vi "Day12-create_map.vi"(11 "string array":string[](array[string])) -> (3 "Map":map{string, string[]}(c390))   [LabVIEW 2021]
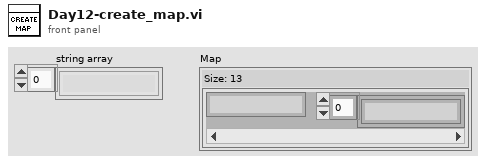
[diagram p1: front panel]
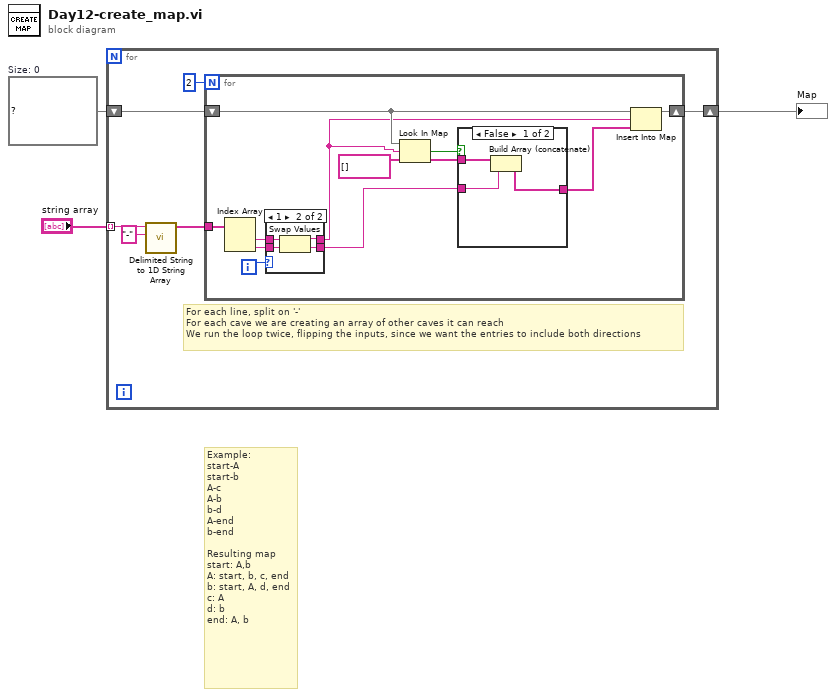
[diagram p0: block diagram]
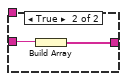
[diagram p3: hidden frame]
diagram:
  w2 = map{string, string[]} {}  # Size: 0
  # "Example:\nstart-A\nstart-b\nA-c\nA-b\nb-d\nA-end\nb-end\n\nResulting map\nstart: A,b\nA: start, b, c, end\nb: start, A, d, end\nc: A\nd: b\nend: A, b"
  n1 = for {
    tunnel: "string array" -> [w9] mode=indexing
    shift-right: [w6] -> w3
    shift-left: w2 -> [w7]
    # "For each line, split on '-'\nFor each cave we are creating an array of other caves it can reach\nWe run the loop twice, flipping the inputs, since we want the entries to include both directions"
    n2 = call <vilib>:"Delimited String to 1D String Array.vi"("delimiter"="-", "delimited string"=w9) -> ("string array"=w5:string[])  [unwired: 9 in]
    n3 = for {
      N: 2 -> [_]
      shift-right: [w17] -> w6
      shift-left: w7 -> [w18]
      tunnel: w5 -> [w15]
      i -> [w14]
      n4 = Index Array(array=w15) -> (element #1=w13:string, element #2=w11:string)  [unwired: 2 in]
      n5 = case shown="1" w14 {
        tunnel: w13 -> [w23 w27]
        tunnel: [w23 w25] -> w12
        tunnel: w11 -> [w22 w26]
        tunnel: [w22 w24] -> w10
        frame 0, Default {
        }
        frame 1 {
          n6 = Swap Values(12:w27, 14:w26) -> (1:w25:string, 3:w24:string)  [unwired: 1 in]
        }
      }
      n7 = Look In Map(map=w18, key=w12, default value=string[] []) -> (key not found?=w20:bool, value=w19:string[])
      n8 = case shown="False" w20 {
        tunnel: w10 -> [w29 w32]
        tunnel: w19 -> [w30 _]
        tunnel: [w28 w31] -> w16
        frame False {
          n9 = Build Array (concatenate)(w30, w29) -> (w28:string[])
        }
        frame True {
          n10 = Build Array(w32) -> (w31:string[])
        }
      }
      n11 = Insert Into Map(map in=w18, key=w12, value=w16) -> (map out=w17:map{string, string[]})  [unwired: 2 out]
    }
  }
  "Map" <- w3
